vi "Send.vi"(8 "error in (no error)":errorcluster, 10 "Message":refnum<class "MSG.lvclass">, 11 "ObserverSet":refnum<class "ObserverSet.lvclass">) -> (0 "error out":errorcluster, 3 "ObserverSet":refnum<class "ObserverSet.lvclass">)   [LabVIEW 2011, in "Messenging.lvlib" / "ObserverSet.lvclass"]
uses:
  ObserverSet.lvclass
  SendOnly/Observer.lvclass
  Message Translation/Translator/Translator.lvclass
  Send/Send.lvclass
  TextVarientMessage/MSG.lvclass
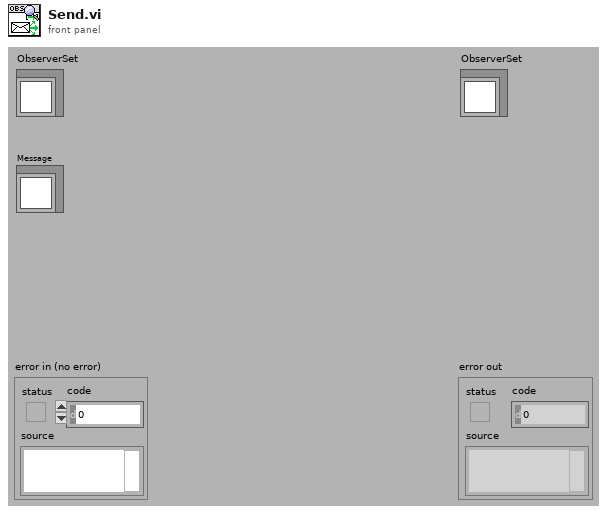
[diagram p1: front panel]
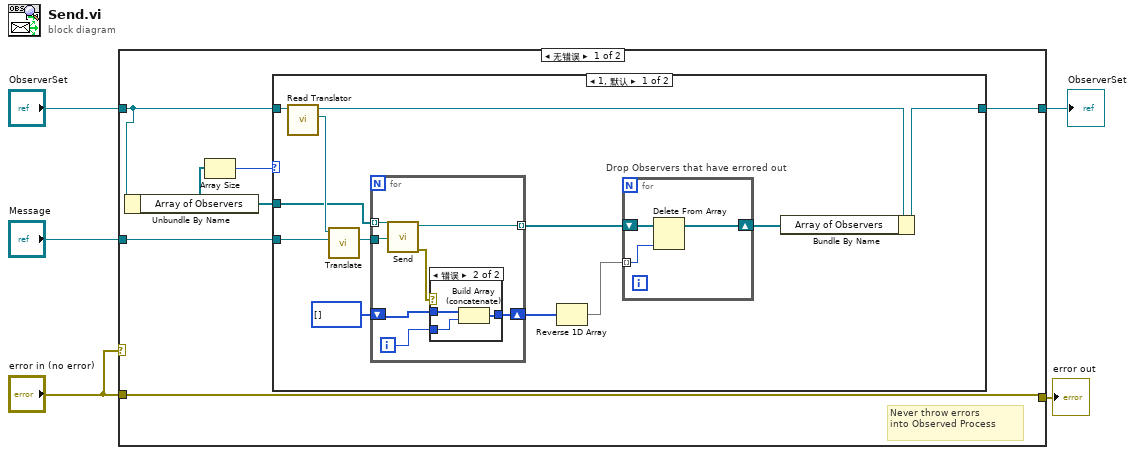
[diagram p0: block diagram]
diagram:
  n1 = case shown="无错误" "error in (no error)" {
    tunnel: "Message" -> [w10 _]
    tunnel: "error in (no error)" -> [w9 w39]
    tunnel: "ObserverSet" -> [w8 w40]
    tunnel: [w9 w39] -> w3
    tunnel: [w11 w40] -> w1
    frame No Error {
      # "Never throw errors\ninto Observed Process"
      n2 = Unbundle By Name(w8) -> ("Array of Observers"=w7:refnum<class "Send.lvclass">[])
      n3 = Array Size(array=w7) -> (size(s)=w6:i32)
      n4 = case shown="1, 默认" w6 {
        tunnel: [w23 w38] -> w11
        tunnel: w10 -> [w21 _]
        tunnel: w8 -> [w17 w38]
        tunnel: w7 -> [w16 _]
        frame 1, Default {
          n5 = call "Read Translator.vi"("Observer.lvclass in"=w17) -> ("Messenging.lvlib:Translator.lvclass"=w22:refnum<class "Translator.lvclass">, "Observer.lvclass out"=w18:refnum<class "ObserverSet.lvclass">)  [unwired: 1 in, 8 out]
          n6 = call-dynamic "Translate.vi"("Message In"=w21, "Translator in"=w22) -> ("Translated Message"=w20:refnum<class "MSG.lvclass">)  [unwired: 9 out]
          n7 = for {
            tunnel: w16 -> [w33] mode=indexing
            tunnel: w20 -> [w32]
            tunnel: [w31] -> w19 mode=indexing
            shift-right: [w29] -> w14
            shift-left: i32[] [] -> [w27]
            i -> [w28]
            n8 = call-dynamic "Send.vi"("Message"=w32, "MSR Parent in"=w33) -> ("error out"=w30:errorcluster, "MSR Parent out"=w31:refnum<class "Send.lvclass">)  [unwired: 1 in, 7 out]
            n9 = case shown="错误" w30 {
              tunnel: [w34 w37] -> w29
              tunnel: w28 -> [_ w36]
              tunnel: w27 -> [w34 w35]
              frame No Error {
              }
              frame Error {
                n10 = Build Array (concatenate)(w35, w36) -> (w37:i32[])
              }
            }
          }
          n11 = Reverse 1D Array(array=w14) -> (reversed array=w12:i32[])
          n12 = for "Drop Observers that have errored out" {
            shift-right: [w25] -> w13
            shift-left: w19 -> [w26]
            tunnel: w12 -> [w24] mode=indexing
            n13 = Delete From Array(array=w26, index=w24) -> (array with subset deleted=w25:refnum<class "Send.lvclass">[])  [unwired: 1 in, 1 out]
          }
          n14 = Bundle By Name(cluster=w18, "Array of Observers"=w13) -> (w23:refnum<class "ObserverSet.lvclass">)
        }
        frame 0 {
        }
      }
    }
    frame Error {
    }
  }
  "error out" <- w3
  "ObserverSet" <- w1
